vi "Read and Update Key (Boolean).vi"(6 "create if not exists (T)":bool=TRUE, 7 "section":string, 8 "error in (no error)":errorcluster, 9 "default":bool, 10 "key":string, 11 "refnum in":T1) -> (0 "error out":errorcluster, 1 "value":bool, 3 "refnum out":T1)   [LabVIEW 2016, in "User Interface.lvlib" / "User Interface.lvclass"]
uses:
  User Interface.lvclass
  <vilib>/Utility/config.llb/Config Data RefNum.ctl
  <vilib>/Utility/config.llb/Read Key (Boolean).vi
  <vilib>/Utility/config.llb/Write Key (Boolean).vi
  <vilib>/Utility/config.llb/NI_LVConfig.lvlib
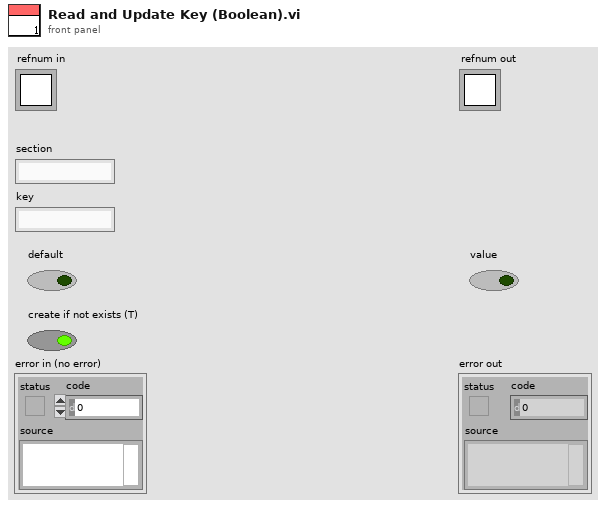
[diagram p1: front panel]
types:
  T1 = typedef "NI_LVConfig.lvlib/Config Data RefNum.ctl" = refnum<k1>
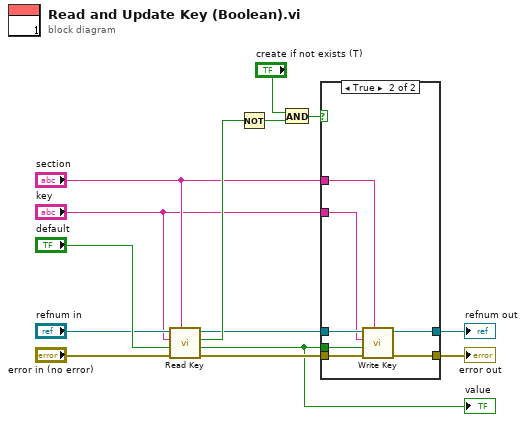
[diagram p0: block diagram]
diagram:
  n1 = call-poly <vilib>:"Read Key.vi"("section"="section", "error in (no error)"="error in (no error)", "default value"="default", "key"="key", "refnum"="refnum in") -> ("error out"=w8:errorcluster, "value"=w1:bool, "found?"=w10:bool, "refnum out"=w9:T1)  [unwired: 3 in]
  "value" <- w1
  n2 = Not(x=w10) -> (.not. x?=w3:bool)
  n3 = And(x="create if not exists (T)", y=w3) -> (x .and. y?=w11:bool)
  n4 = case shown="True" w11 {
    tunnel: w9 -> [w16 w23]
    tunnel: w8 -> [w15 w22]
    tunnel: [w15 w21] -> w7
    tunnel: [w16 w20] -> w6
    tunnel: w1 -> [_ w17]
    tunnel: "section" -> [_ w19]
    tunnel: "key" -> [_ w18]
    frame False {
    }
    frame True {
      n5 = call-poly <vilib>:"Write Key.vi"("section"=w19, "error in (no error)"=w22, "value"=w17, "key"=w18, "refnum"=w23) -> ("error out"=w21:errorcluster, "refnum out"=w20:T1)  [unwired: 4 in, 1 out]
    }
  }
  "error out" <- w7
  "refnum out" <- w6
